vi "AlliGator Remove Keywords from Action String.vi"(8 "error in (no error)":errorcluster, 11 "String":string) -> (0 "error out":errorcluster, 3 "String w/o keywords":string)   [LabVIEW 2021, in "AlliGator Notebook.lvlib"]
doc: "Removes frequent internal events from list of printed events in verbose mode."
uses:
  AlliGator Notebook.lvlib
panel:
  # "see the AlliGator License on the block diagram (Ctrl+E or Window:Show Block Diagram)"
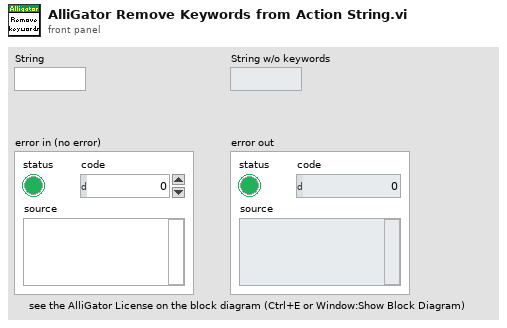
[diagram p1: front panel]
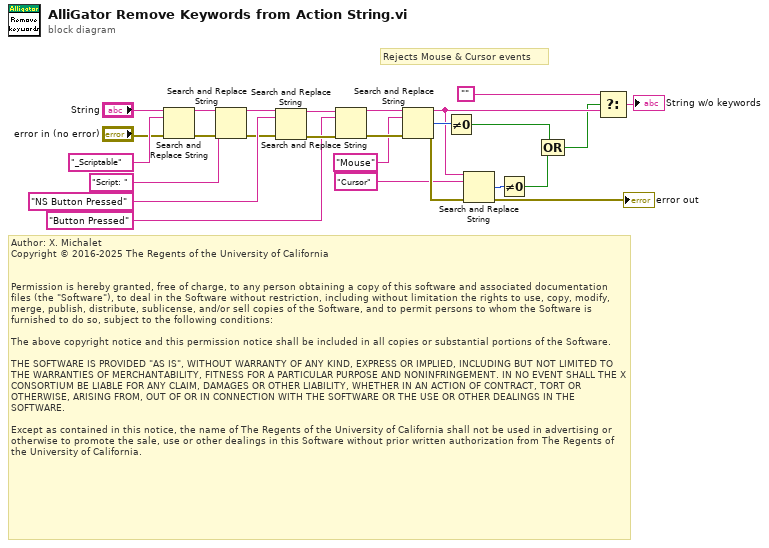
[diagram p0: block diagram]
diagram:
  # "Author: X. Michalet\nCopyright © 2016-2025 The Regents of the University of California\n \n\nPermission is hereby granted, free of charge, to any person obtaining a copy of this software and associated documentation files (the \"Software\"), to deal in the Software without restriction, including without limitation the rights to use, copy, modify, merge, publish, distribute, sublicense, and/or sell copies of the Software, and to permit persons to whom the Software is furnished to do so, subject to the following conditions:\n\nThe above copyright notice and this permission notice shall be included in all copies or substantial portions of the Software.\n\nTHE SOFTWARE IS PROVIDED \"AS IS\", WITHOUT WARRANTY OF ANY KIND, EXPRESS OR IMPLIED, INCLUDING BUT NOT LIMITED TO THE WARRANTIES OF MERCHANTABILITY, FITNESS FOR A PARTICULAR PURPOSE AND NONINFRINGEMENT. IN NO EVENT SHALL THE X CONSORTIUM BE LIABLE FOR ANY CLAIM, DAMAGES OR OTHER LIABILITY, WHETHER IN AN ACTION OF CONTRACT, TORT OR OTHERWISE, ARISING FROM, OUT OF OR IN CONNECTION WITH THE SOFTWARE OR THE USE OR OTHER DEALINGS IN THE SOFTWARE.\n\nExcept as contained in this notice, the name of The Regents of the University of California shall not be used in advertising or otherwise to promote the sale, use or other dealings in this Software without prior written authorization from The Regents of the University of California."
  # "Rejects Mouse & Cursor events"
  n1 = Search and Replace String(input string="String", search string="_Scriptable" ("substring (\"\")"), error in="error in (no error)") -> (result string=w24:string, error out=w25:errorcluster)  [unwired: 5 in, 2 out]
  n2 = Search and Replace String(input string=w24, search string="Script: " ("substring (\"\")"), error in=w25) -> (result string=w17:string, error out=w18:errorcluster)  [unwired: 5 in, 2 out]
  n3 = Search and Replace String(input string=w17, search string="NS Button Pressed" ("substring (\"\")"), error in=w18) -> (result string=w19:string, error out=w20:errorcluster)  [unwired: 5 in, 2 out]
  n4 = Search and Replace String(input string=w19, search string="Button Pressed" ("substring (\"\")"), error in=w20) -> (result string=w13:string, error out=w14:errorcluster)  [unwired: 5 in, 2 out]
  n5 = Search and Replace String(input string=w13, search string="Mouse", error in=w14) -> (result string=w6:string, number of replacements=w11:i32, error out=w7:errorcluster)  [unwired: 5 in, 1 out]
  n6 = Not Equal To 0?(x=w11) -> (x != 0?=w10:bool)
  n7 = Search and Replace String(input string=w6, search string="Cursor", error in=w7) -> (number of replacements=w4:i32, error out=→"error out":errorcluster)  [unwired: 5 in, 2 out]
  n8 = Not Equal To 0?(x=w4) -> (x != 0?=w1:bool)
  n9 = Compound Arithmetic op=OR(w10, w1) -> (w3:bool)
  n10 = Select(t="", s=w3, f=w6) -> (s? t:f=→"String w/o keywords":string)
